vi "PH_IEEE1394Camera.calculate serial number.vi"(1 "SerialNumberLow":u32, 2 "SerialNumberHigh":u32) -> (0 "Serial Number":dbl)   [LabVIEW 2014, in "PH_IEEE1394Camera.lvlib"]
uses:
  PH_IEEE1394Camera.lvlib
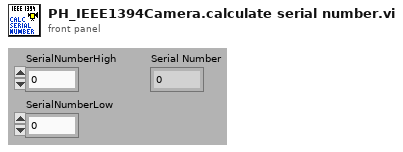
[diagram p1: front panel]
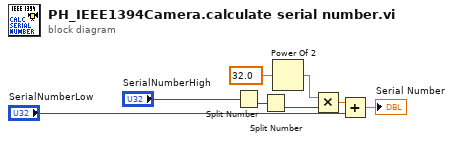
[diagram p0: block diagram]
diagram:
  n1 = Split Number(x="SerialNumberHigh") -> (lo(x)=w4:u16)  [unwired: 1 out]
  n2 = Split Number(x=w4) -> (lo(x)=w5:u8)  [unwired: 1 out]
  n3 = Power Of 2(x=32.0) -> (2^x=w2:dbl)
  n4 = Multiply(x=w2, y=w5) -> (x*y=w3:dbl)
  n5 = Add(x=w3, y="SerialNumberLow") -> (x+y=→"Serial Number":dbl)
